vi "First Step.vi"(8 "error in (no error)":errorcluster, 11 "Continuous.lvclass in":refnum<class "Continuous.lvclass">) -> (0 "error out":errorcluster, 2 "Current Position":dbl, 3 "Continuous.lvclass out":refnum<class "Continuous.lvclass">)   [LabVIEW 2009, in "Continuous.lvclass"]
uses:
  Continuous.lvclass
  Instruments/Magnet/Power Supply/Power Supply.lvclass
  Scanner/Scanner.lvclass
  Continuous.lvclass/Continuous.ctl
  Instruments/Magnet/Power Supply/Ramping Mode.ctl
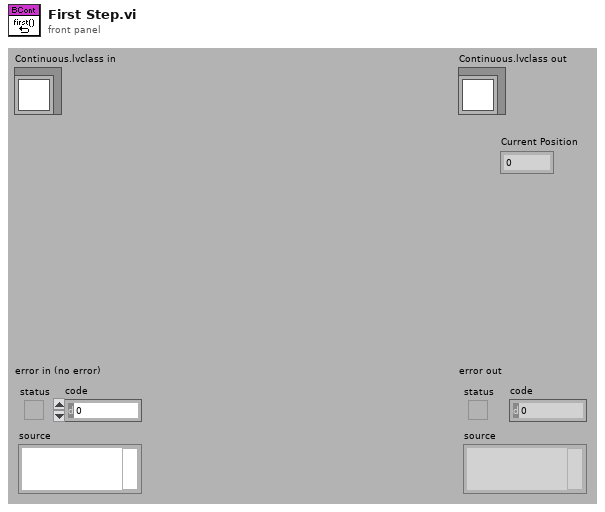
[diagram p1: front panel]
types:
  T1 = typedef "Scanner.lvclass/Range.ctl" = cluster{"xi":dbl, "xf":dbl, "dx":dbl, "Return to...?":bool, "Return to":dbl}
  T2 = typedef "Power Supply.lvclass/Ramping Mode.ctl" = enum16{"Train Speed", "Maximum Speed", "Manual"}
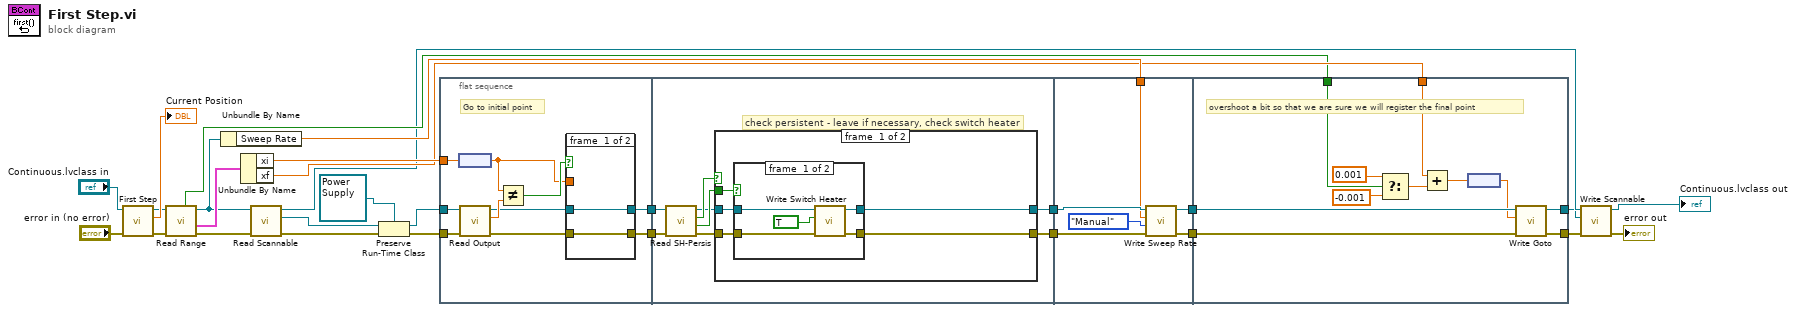
[diagram p0: block diagram]
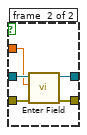
[diagram p2: hidden frame]
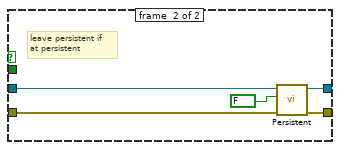
[diagram p4: hidden frame]
diagram:
  n1 = call-parent "First Step.vi"("error in (no error)"="error in (no error)", "Scanner.lvclass in"="Continuous.lvclass in") -> ("error out"=w23:errorcluster, "Current Position"=→"Current Position":dbl, "Scanner.lvclass out"=w25:refnum<class "Continuous.lvclass">)  [unwired: 7 out]
  n2 = call-dynamic "Read Range.vi"("error in (no error)"=w23, "Scanner.lvclass in"=w25) -> ("error out"=w6:errorcluster, "Range"=w24:T1, "Scanner.lvclass out"=w3:refnum<class "Continuous.lvclass">, "Scanning Up?"=w14:bool)  [unwired: 6 out]
  n3 = Unbundle By Name(w3) -> ("Sweep Rate"=w21:dbl[unit])
  n4 = Unbundle By Name(w24) -> ("xi"=w22:dbl, "xf"=w17:dbl)
  n5 = call-dynamic "Read Scannable.vi"("error in (no error)"=w6, "Scanner.lvclass in"=w3) -> ("error out"=w7:errorcluster, "Scannable.lvclass"=w11:refnum<class "Scannable.lvclass">, "Scanner.lvclass out"=w12:refnum<class "Continuous.lvclass">)  [unwired: 7 in]
  n6 = Preserve Run-Time Class(object in=w11, error in=w7, 2:refnum<class "Power Supply.lvclass"> refnum ("Power Supply in")) -> (object out=w9:refnum<class "Power Supply.lvclass">, error out=w8:errorcluster)
  n7 = flat-sequence {
    tunnel: w22 -> [w36]
    tunnel: [w35] -> w20
    tunnel: [w33] -> w15
    tunnel: w9 -> [w30]
    tunnel: w8 -> [w29]
    tunnel: w20 -> [w51]
    tunnel: [w49] -> w19
    tunnel: [w48] -> w16
    tunnel: w15 -> [w46]
    tunnel: w21 -> [w74]
    tunnel: w19 -> [w76]
    tunnel: [w75] -> w18
    tunnel: w16 -> [w72]
    tunnel: [w71] -> w13
    tunnel: w18 -> [w84]
    tunnel: w17 -> [w82]
    tunnel: w14 -> [w81]
    tunnel: w13 -> [w79]
    tunnel: [w78] -> w2
    tunnel: [w77] -> w1
    frame #0 {
      # "Go to initial point"
      n8 = node(w36) -> (w31:dbl[unit])
      n9 = call-dynamic "Read Output.vi"("error in (no error)"=w29, "Power Supply in"=w30) -> ("error out"=w32:errorcluster, "Field"=w38:dbl[unit], "Power Supply out"=w34:refnum<class "Power Supply.lvclass">)  [unwired: 6 in, 1 out]
      n10 = Not Equal?(x=w31, y=w38) -> (x != y?=w37:bool)
      n11 = case shown="True" w37 {
        tunnel: w31 -> [_ w41]
        tunnel: [w40 w45] -> w35
        tunnel: w34 -> [w40 w44]
        tunnel: [w39 w43] -> w33
        tunnel: w32 -> [w39 w42]
        frame #0 {
        }
        frame #1 {
          n12 = call-dynamic "Enter Field.vi"("error in (no error)"=w42, "Target field"=w41, "Power Supply in"=w44) -> ("error out"=w43:errorcluster, "Power Supply out"=w45:refnum<class "Power Supply.lvclass">)  [unwired: 7 in]
        }
      }
    }
    frame #1 {
      # "check persistent - leave if necessary, check switch heater"
      n13 = call-dynamic "Read SH-Persis.vi"("error in (no error)"=w46, "Power Supply in"=w51) -> ("error out"=w47:errorcluster, "SHon?"=w53:bool, "pers?"=w52:bool, "Power Supply out"=w50:refnum<class "Power Supply.lvclass">)  [unwired: 4 in, 2 out]
      n14 = case shown="True" w52 {
        tunnel: w53 -> [w58 _]
        tunnel: w50 -> [w56 w69]
        tunnel: [w55 w68] -> w49
        tunnel: [w54 w67] -> w48
        tunnel: w47 -> [w57 w66]
        frame #0 {
          n15 = case shown="False" w58 {
            tunnel: w57 -> [w63 w65]
            tunnel: w56 -> [w62 w64]
            tunnel: [w61 w64] -> w55
            tunnel: [w60 w65] -> w54
            frame #0 {
              n16 = call-dynamic "Write Switch Heater.vi"("error in (no error)"=w63, "Turn SH On?"=TRUE, "Power Supply in"=w62) -> ("error out"=w60:errorcluster, "Power Supply out"=w61:refnum<class "Power Supply.lvclass">)  [unwired: 7 in]
            }
            frame #1 {
            }
          }
        }
        frame #1 {
          # "leave persistent if\nat persistent"
          n17 = call-dynamic "Persistent.vi"("error in (no error)"=w66, "Go to persistent mode?"=FALSE, "Power Supply in"=w69) -> ("error out"=w67:errorcluster, "Power Supply out"=w68:refnum<class "Power Supply.lvclass">)  [unwired: 7 in]
        }
      }
    }
    frame #2 {
      n18 = call-dynamic "Write Sweep Rate.vi"("error in (no error)"=w72, "Ramping Mode"=Ramping_Mode."Manual", "rate"=w74, "Power Supply in"=w76) -> ("error out"=w71:errorcluster, "Power Supply out"=w75:refnum<class "Power Supply.lvclass">)  [unwired: 6 in]
    }
    frame #3 {
      # "overshoot a bit so that we are sure we will register the final point"
      n19 = Select(t=0.001, s=w81, f=-0.001) -> (s? t:f=w87:dbl)
      n20 = Add(x=w82, y=w87) -> (x+y=w83:dbl)
      n21 = node(w83) -> (w80:dbl[unit])
      n22 = call-dynamic "Write Goto.vi"("error in (no error)"=w79, "Target"=w80, "Power Supply in"=w84) -> ("error out"=w77:errorcluster, "Power Supply out"=w78:refnum<class "Power Supply.lvclass">)  [unwired: 7 in]
    }
  }
  n23 = call-dynamic "Write Scannable.vi"("error in (no error)"=w1, "Scannable.lvclass"=w2, "Scanner.lvclass in"=w12) -> ("error out"=→"error out":errorcluster, "Scanner.lvclass out"=→"Continuous.lvclass out":refnum<class "Continuous.lvclass">)  [unwired: 7 in]
